vi "init.vi"(8 "error in (no error)":errorcluster, 11 "Logger in":refnum<class "StiffnessLog.lvclass">) -> (0 "error out":errorcluster, 3 "Logger out":refnum<class "StiffnessLog.lvclass">)   [LabVIEW 2013, in "StiffnessLog.lvclass"]
uses:
  StiffnessLog.lvclass
  <userlib>/Common/Log/Config/Log.ctl
  <userlib>/Common/Log/Log/Log.lvclass/Log.ctl
  ConfigurationThisComponent/ConfigurationThisComponent.lvclass
  <userlib>/Common/Log/Log/Log.lvclass
  <userlib>/Common/Log/Log.lvlib
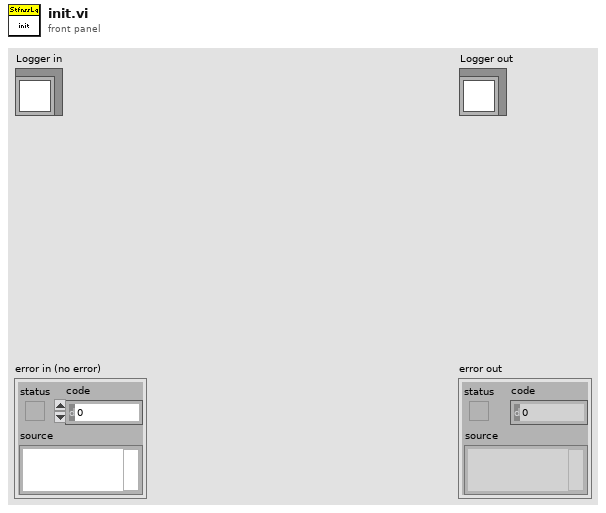
[diagram p1: front panel]
types:
  T1 = typedef "Log.lvlib/Log.ctl" = cluster{"Log Directory":path, "Log Filename Base":string, "Max records per file":u32, "Comment":string}
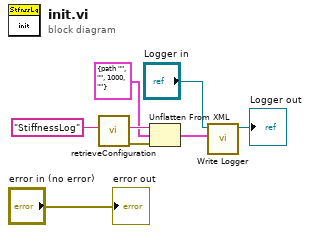
[diagram p0: block diagram]
diagram:
  n1 = call "retrieveConfiguration.vi"("configName"="StiffnessLog") -> ("error out"=w6:errorcluster, "xmlConfig"=w7:string)  [unwired: 8 in, 1 out]
  n2 = Unflatten From XML(xml string=w7, type=T1 {"Log Directory"=path "", "Log Filename Base"="", "Max records per file"=1000, "Comment"=""} ("Logger"), error in (no error)=w6) -> (value=w3:T1)  [unwired: 1 out]
  n3 = call <userlib>:"Write Logger.vi"("Logger"=w3, "Logger in"="Logger in") -> ("Logger out"=→"Logger out":refnum<class "StiffnessLog.lvclass">)  [unwired: 9 in]
  "error out" <- "error in (no error)"
